vi "Main.vi"(11 "Module Admin":refnum<class "Delacor_lib_QMH_Cloneable Module Admin.lvclass">) -> ()   [LabVIEW 2020, in "Arduino-Adafruit stepper.lvlib"]
doc: "This template is based off of the Queued Message Handler design pattern and the Queued Message Handler project template that ships with LabVIEW.\n\nThe main difference is that the queue is private to this module and communication between modules is performed via Broadcast and Request events.\n\nRequest events are wrapped in public API methods and are handled in the Event Handling Loop (EHL) of this VI. Any module can register for Broadcast events sent by this module. The EHL generates messages based on user interface actions.\n\nThe Message Handling Loop (MHL) processes messages generated by the EHL, or by other messages. The messages are string values, so new messages can be added easily to the Message Cases case structure in the MHL. Each message cluster can also provide an optional value for Message Data, which is a variant that can be converted to whatever message-specific data is required.\n_____\nBased on DQMH Project Template 7.0.1.1316."
uses:
  Arduino-Adafruit stepper.lvlib
  <vilib>/Delacor/Delacor QMH/Libraries/Cloneable Module Admin_class/Delacor_lib_QMH_Cloneable Module Admin.lvclass
  C:/Program Files (x86)/National Instruments/LabVIEW 2020/vi.lib/Delacor/Delacor QMH/Libraries/Module Admin_class/Delacor_lib_QMH_Module Admin.lvclass
  Module Data--cluster.ctl
  <vilib>/Delacor/Delacor QMH/Libraries/Cloneable Module Admin_class/Delacor_lib_QMH_Cloneable Module Admin.lvclass/Delacor_lib_QMH_Cloneable Module Admin.ctl
  Stop Argument--cluster.ctl
  <vilib>/Delacor/Delacor QMH/Libraries/Message Queue_class/Delacor_lib_QMH_Message Queue.lvclass/Delacor_lib_QMH_Message Queue.ctl
  <vilib>/Delacor/Delacor QMH/Libraries/Module Admin_class/Delacor_lib_QMH_Module Admin.lvclass/Delacor_lib_QMH_Module Admin.ctl
  Connect Argument--cluster.ctl
  Arduino stepper library/Public/Controls/Com Port Options.ctl
  Disconnect Argument--cluster.ctl
  Init motors Argument--cluster.ctl
  Arduino stepper library/Public/Controls/Motor initialization parameters--cluster.ctl
  Home motors Argument--cluster.ctl
  Arduino stepper library/Public/Controls/Motor direction.ctl
  <vilib>/Utility/miscctls.llb/LVPointTypeDef.ctl
  <vilib>/Instr/_visa.llb/VISA Flush IO Buffer Mask.ctl
  <vilib>/Instr/_visa.llb/VISA Set IO Buffer Mask.ctl
  <vilib>/Delacor/Delacor QMH/Libraries/Cloneable Module Admin_class/Delacor_lib_QMH_Get Module ID.vi
  <vilib>/Delacor/Delacor QMH/Libraries/Message Queue_class/Delacor_lib_QMH_Enqueue Message (Single).vi
  <vilib>/Delacor/Delacor QMH/Libraries/Module Admin_class/Delacor_lib_QMH_Get External Launch.vi
  <vilib>/Instr/_visa.llb/VISA Configure Serial Port (Instr).vi
  <vilib>/Delacor/Delacor QMH/Libraries/Message Queue_class/Delacor_lib_QMH_Message Queue.lvclass
  Arduino stepper library/Control de MaP.lvlib
panel:
  out "error out":errorcluster
  out "Status":string
  # "Other processes communicate with this Module via its Public API (wrappers for its Request Events).\n\nThis Module communicates with other processes via its Broadcast Events.\nAny process that wants to receive these messages can register for this module's Broadcast events."
  # "This template is for the DQMH framework. See the block diagram for more information on how to use this template."
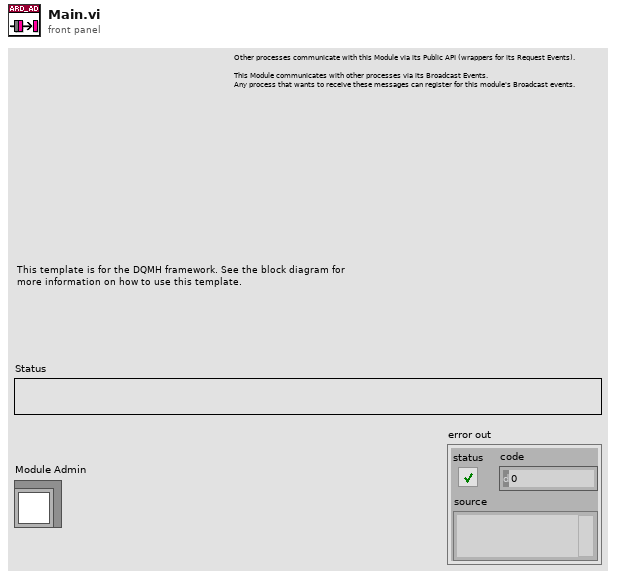
[diagram p1: front panel]
types:
  T1 = typedef "Arduino-Adafruit stepper.lvlib/Request Events--cluster.ctl" = cluster{"Stop Module":refnum<user-event>, "Show Panel":refnum<user-event>, "Hide Panel":refnum<user-event>, "Show Diagram":refnum<user-event>, "Get Module Execution Status":refnum<user-event>, "Initialize Arduino":refnum<user-event>, "Connect":refnum<user-event>, "Disconnect":refnum<user-event>, "Init motors":refnum<user-event>, "Home motors":refnum<user-event>}
  T2 = typedef "Arduino-Adafruit stepper.lvlib/Module Data--cluster.ctl" = cluster{"Status":string, "VISA resource":refnum<visa-resource-name>, "Connected?":bool}
  T3 = enum32{"invalid lock state", "Not Locked", "Locked (No Password)", "Password-protected"}
  T4 = typedef "Arduino-Adafruit stepper.lvlib/Stop Argument--cluster.ctl" = cluster{"Module ID":i32, "Origin":string, "Exit via Stop Module Req?":bool, "Wait for Module to stop?":bool}
  T5 = typedef "Arduino-Adafruit stepper.lvlib/Connect Argument--cluster.ctl" = cluster{"Module ID":i32, "VISA resource":refnum<visa-resource-name>, "COM options":T6}
  T6 = typedef "Control de MaP.lvlib/Com Port Options.ctl" = cluster{"baud rate":u32, "data bits":u16, "parity":enum16{"None", "Odd", "Even", "Mark", "Space"}}
  T7 = typedef "Arduino-Adafruit stepper.lvlib/Disconnect Argument--cluster.ctl" = cluster{"Module ID":i32, "Boolean":bool}
  T8 = typedef "Arduino-Adafruit stepper.lvlib/Init motors Argument--cluster.ctl" = cluster{"Module ID":i32, "Comando":T9}
  T9 = typedef "Control de MaP.lvlib/Motor initialization parameters--cluster.ctl" = cluster{"Action":u8, "Steps per rev motor 1":u8, "Steps per rev motor 2":u8, "RPM motor 1":u16, "RPM motor 2":u16}
  T10 = typedef "Arduino-Adafruit stepper.lvlib/Home motors Argument--cluster.ctl" = cluster{"Module ID":i32, "Home direction (M1)":T11, "Home direction (M2)":T11}
  T11 = typedef "Control de MaP.lvlib/Motor direction.ctl" = u8
  T12 = typedef "LVPointTypeDef.ctl" = cluster{"Horizontal":i16, "Vertical":i16}
  T13 = enum32{"Invalid", "Standard", "Closed", "Hidden", "Minimized", "Maximized"}
  T14 = typedef "VISA Set IO Buffer Mask.ctl" = u16
  T15 = typedef "VISA Flush IO Buffer Mask.ctl" = u16
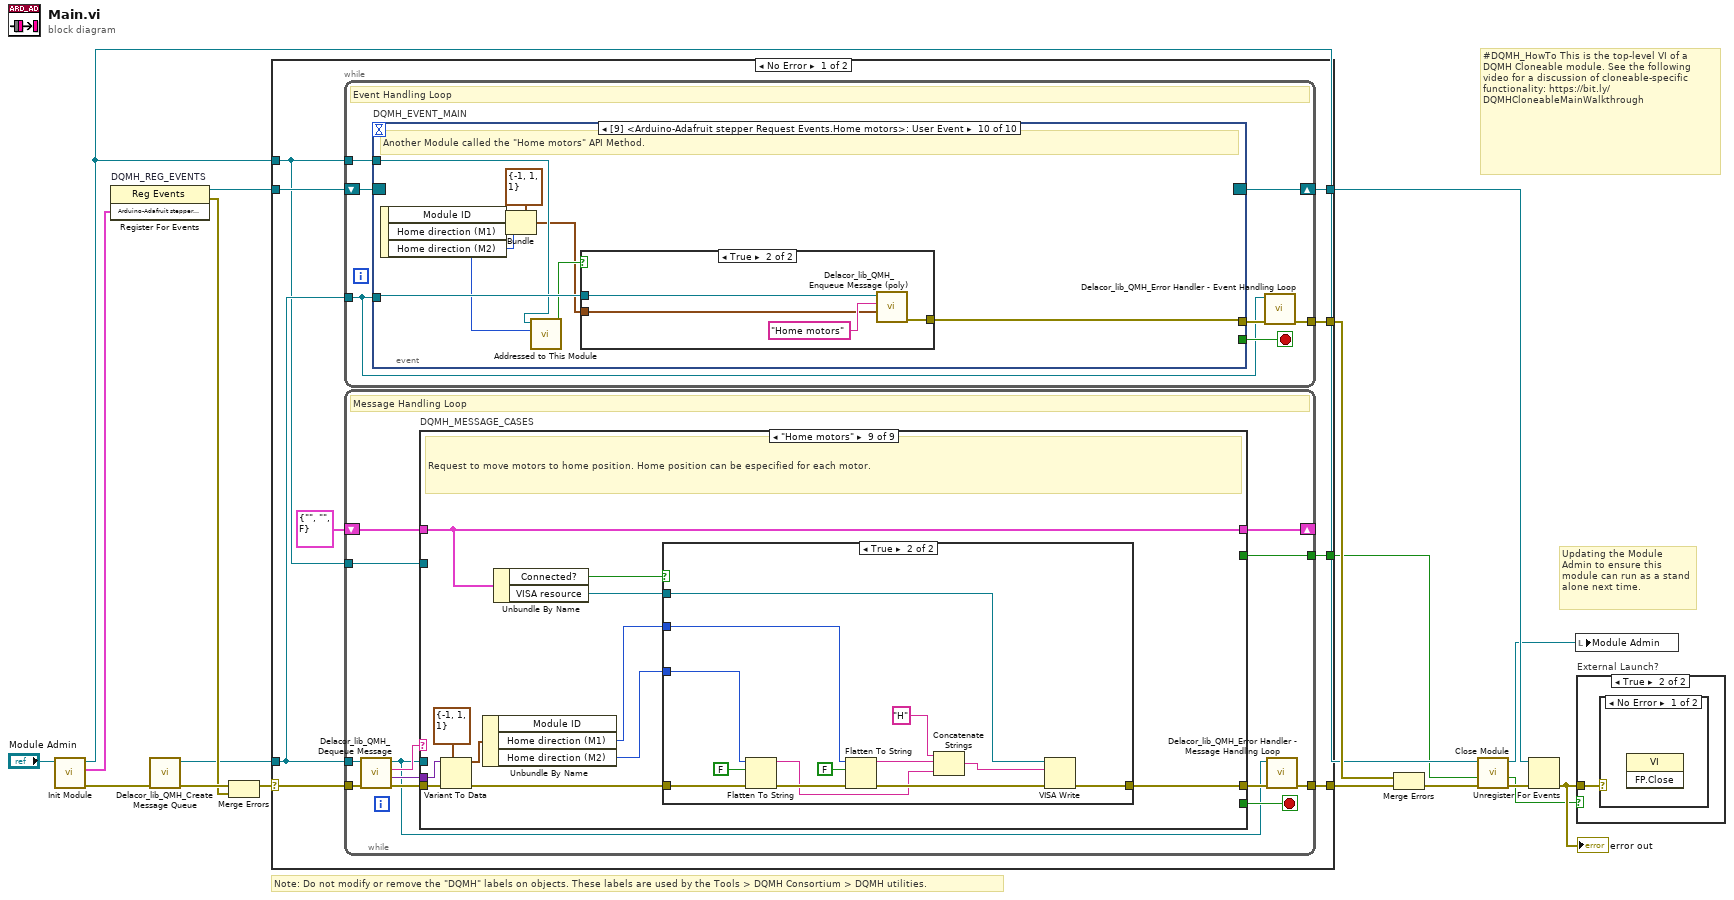
[diagram p0: block diagram]
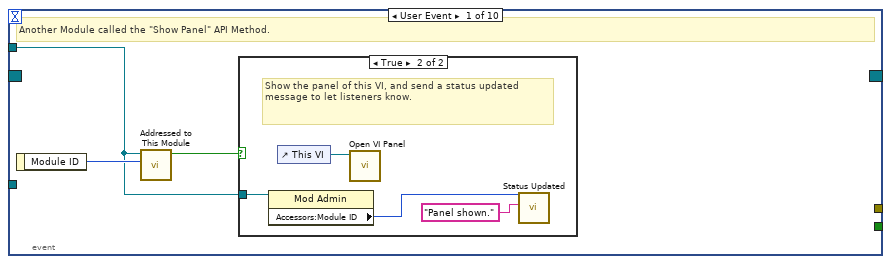
[diagram p2: hidden frame]
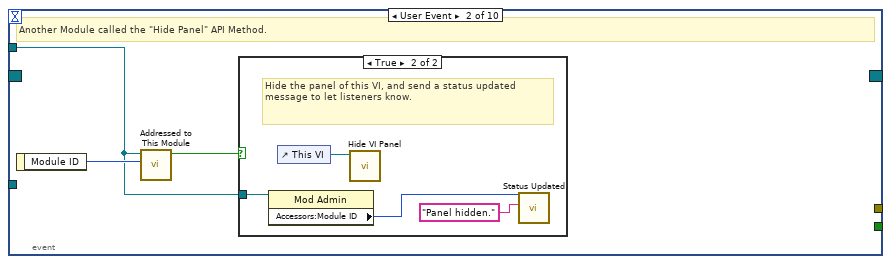
[diagram p4: hidden frame]
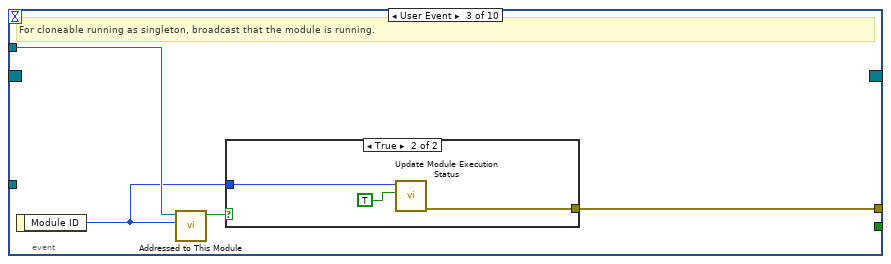
[diagram p6: hidden frame]
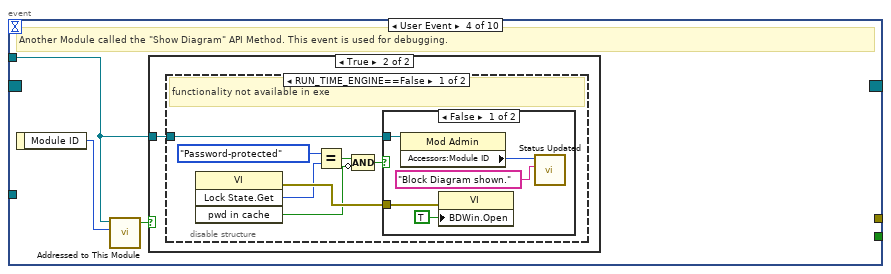
[diagram p8: hidden frame]
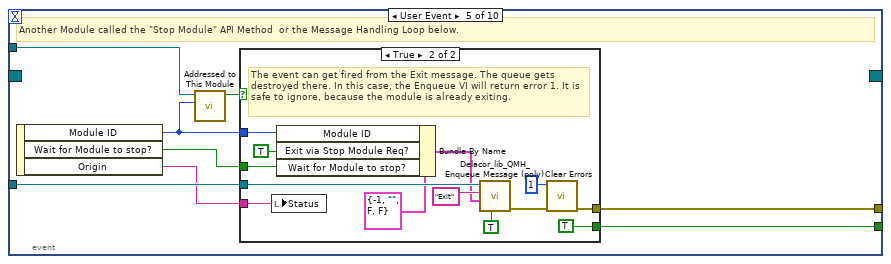
[diagram p12: hidden frame]
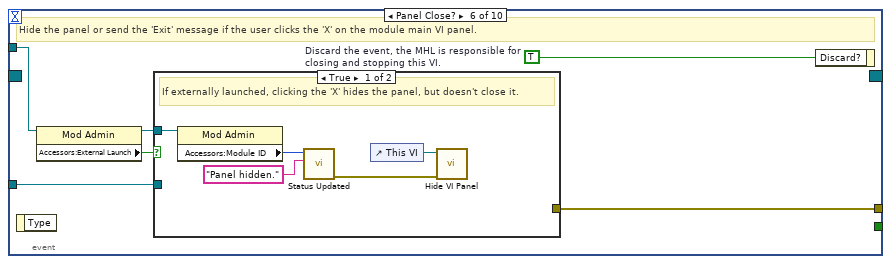
[diagram p14: hidden frame]
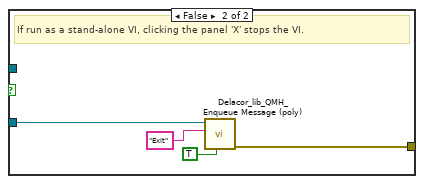
[diagram p15: hidden frame]
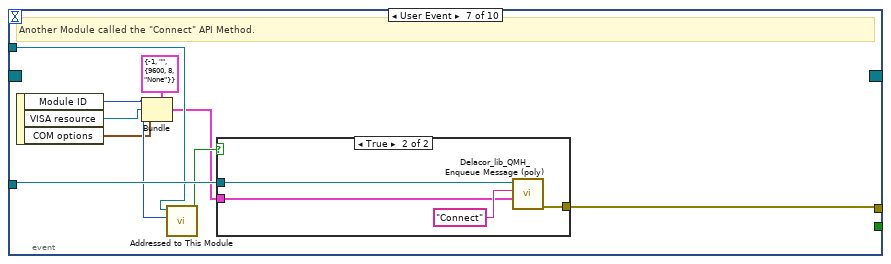
[diagram p16: hidden frame]
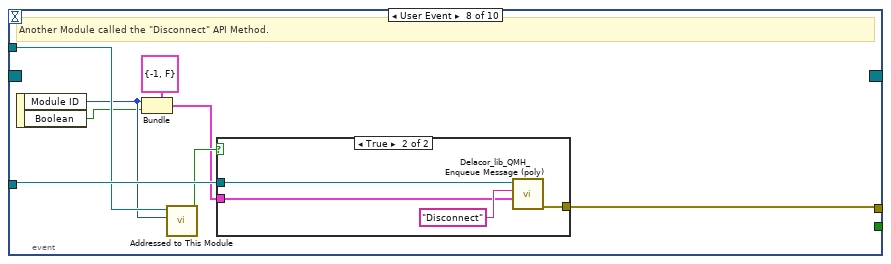
[diagram p18: hidden frame]
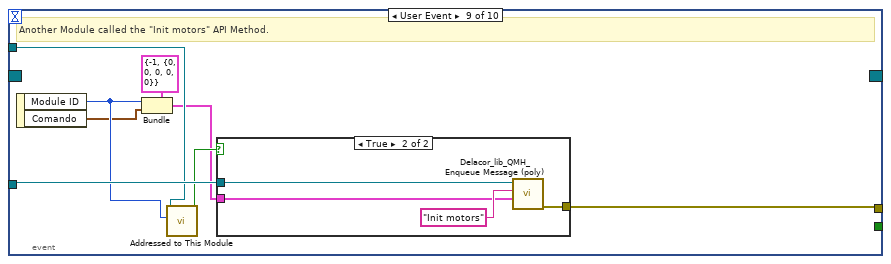
[diagram p20: hidden frame]
diagram:
  # "#DQMH_HowTo This is the top-level VI of a DQMH Cloneable module. See the following video for a discussion of cloneable-specific functionality: https://bit.ly/DQMHCloneableMainWalkthrough"
  # "Note: Do not modify or remove the \"DQMH\" labels on objects. These labels are used by the Tools > DQMH Consortium > DQMH utilities."
  # "Updating the Module Admin to ensure this module can run as a stand alone next time."
  n1 = call "Init Module.vi"("Cloneable Module Admin in"="Module Admin") -> ("error out"=w15:errorcluster, "Arduino-Adafruit stepper Request Events"=w7:T1, "Cloneable Module Admin out"=w4:refnum<class "Delacor_lib_QMH_Cloneable Module Admin.lvclass">)  [unwired: 8 in]
  n2 = register-events "DQMH_REG_EVENTS"(w7) -> (reference out=w8:refnum<event-registration>, error out=w10:errorcluster)  [unwired: 2 in]
  n3 = call <vilib>:"Delacor_lib_QMH_Create Message Queue.vi"("error in"=w15) -> ("error out"=w12:errorcluster, "Message Queue"=w6:refnum<class "Delacor_lib_QMH_Message Queue.lvclass">)  [unwired: 9 in]
  n4 = Merge Errors(w12, w10) -> (w11:errorcluster)
  n5 = case shown="No Error" w11 {
    selector: w11 -> [w25 w401]
    tunnel: [w27 w400] -> w16
    tunnel: [w24 w399] -> w9
    tunnel: w8 -> [w22 w399]
    tunnel: w6 -> [w21 w392]
    tunnel: [w26 _] -> w17
    tunnel: w4 -> [w20 w395]
    tunnel: [w19 _] -> w2
    frame No Error {
      n6 = while {
        tunnel: w21 -> [w28]
        shift-right: [w31] -> w24
        shift-left: w22 -> [w32]
        tunnel: [w33] -> w26
        tunnel: w20 -> [w29]
        stop <- w30 stop-if-true
        # "Event Handling Loop"
        n7 = event "DQMH_EVENT_MAIN" shown="[9] <Arduino-Adafruit stepper Request Events.Home motors>: User Event" {
          selector: w32 -> [_ _ _ _ _ _ _ _ _ _]
          dyn-events: [_ _ _ _ _ _ _ _ _ _] -> w31
          timeout: _ -> [_ _ _ _ _ _ _ _ _ _]
          tunnel: [_ _ _ _ w75 _ _ _ _ _] -> w30
          tunnel: w28 -> [_ _ _ _ w78 w95 w116 w128 w140 w153]
          tunnel: [_ _ w52 _ w79 w98 w108 w121 w134 w145] -> w34
          tunnel: w29 -> [w35 w42 w50 w56 w77 w96 w114 w126 w138 w151]
          event User Event {
            # "Another Module called the \"Show Panel\" API Method."
            n8 = event-data() -> ("Module ID"=w36:i32)  [unwired: 1 in]
            n9 = call "Addressed to This Module.vi"("Module ID from Argument"=w36, "Module Admin"=w35) -> ("Addressed to this instance?"=w37:bool)  [unwired: 8 in, 1 out]
            n10 = case shown="True" w37 {
              tunnel: w35 -> [_ w39]
              frame False {
              }
              frame True {
                # "Show the panel of this VI, and send a status updated message to let listeners know."
                n11 = property on="Property Node" class="Mod Admin"(reference=w39) -> ("Accessors:Module ID"=w38:i32)  [unwired: 1 in, 2 out]
                n12 = control-ref of="This VI"() -> (w41:refnum<vi>)
                n13 = call "Open VI Panel.vi"("VI"=w41) -> ()  [unwired: 10 in, 1 out]
                n14 = call "Status Updated.vi"("Status"="Panel shown." ("format string"), "Module ID"=w38) -> ()  [unwired: 9 in, 1 out]
              }
            }
          }
          event User Event {
            # "Another Module called the \"Hide Panel\" API Method."
            n15 = event-data() -> ("Module ID"=w43:i32)  [unwired: 1 in]
            n16 = call "Addressed to This Module.vi"("Module ID from Argument"=w43, "Module Admin"=w42) -> ("Addressed to this instance?"=w44:bool)  [unwired: 8 in, 1 out]
            n17 = case shown="True" w44 {
              tunnel: w42 -> [_ w46]
              frame False {
              }
              frame True {
                # "Hide the panel of this VI, and send a status updated message to let listeners know."
                n18 = property on="Property Node" class="Mod Admin"(reference=w46) -> ("Accessors:Module ID"=w45:i32)  [unwired: 1 in, 2 out]
                n19 = control-ref of="This VI"() -> (w48:refnum<vi>)
                n20 = call "Hide VI Panel.vi"("VI"=w48) -> ()  [unwired: 10 in, 1 out]
                n21 = call "Status Updated.vi"("Status"="Panel hidden." ("format string"), "Module ID"=w45) -> ()  [unwired: 9 in, 1 out]
              }
            }
          }
          event User Event {
            # "For cloneable running as singleton, broadcast that the module is running."
            n22 = event-data() -> ("Module ID"=w49:i32)  [unwired: 1 in]
            n23 = call "Addressed to This Module.vi"("Module ID from Argument"=w49, "Module Admin"=w50) -> ("Addressed to this instance?"=w51:bool)  [unwired: 8 in, 1 out]
            n24 = case shown="True" w51 {
              tunnel: [_ w55] -> w52
              tunnel: w49 -> [_ w54]
              frame False {
              }
              frame True {
                n25 = call "Update Module Execution Status.vi"("Running?"=TRUE, "Module ID"=w54) -> ("error out"=w55:errorcluster)  [unwired: 9 in]
              }
            }
          }
          event User Event {
            # "Another Module called the \"Show Diagram\" API Method. This event is used for debugging."
            n26 = event-data() -> ("Module ID"=w57:i32)  [unwired: 1 in]
            n27 = call "Addressed to This Module.vi"("Module ID from Argument"=w57, "Module Admin"=w56) -> ("Addressed to this instance?"=w58:bool)  [unwired: 8 in, 1 out]
            n28 = case shown="True" w58 {
              tunnel: w56 -> [_ w59]
              frame False {
              }
              frame True {
                n29 = disable-structure shown="RUN_TIME_ENGINE==False" {
                  disable-tunnel: w59 -> [w60 _]
                  frame condition #0 (active) {
                    # "functionality not available in exe"
                    n30 = invoke on="Invoke Node" class="VI" method="Lock State.Get"() -> (error out=w66:errorcluster, "Get Lock State"=w65:T3, "pwd in cache"=w62:bool)  [unwired: 4 in, 1 out]
                    n31 = Equal?(x=T3."Password-protected", y=w65) -> (x = y?=w63:bool)
                    n32 = Compound Arithmetic op=AND(w63, invert w62) -> (w61:bool)
                    n33 = case shown="False" w61 {
                      tunnel: w66 -> [w71 _]
                      tunnel: w60 -> [w68 _]
                      frame False {
                        n34 = property on="Property Node" class="Mod Admin"(reference=w68) -> ("Accessors:Module ID"=w67:i32)  [unwired: 1 in, 2 out]
                        n35 = property on="Property Node" class="VI"(error in=w71, "BDWin.Open"=TRUE ("Block Diagram Window:Open")) -> ()  [unwired: 1 in, 2 out]
                        n36 = call "Status Updated.vi"("Status"="Block Diagram shown." ("format string"), "Module ID"=w67) -> ()  [unwired: 9 in, 1 out]
                      }
                      frame True {
                        # "Password-protected VI, and the password is not in the cache. Do not show the diagram."
                      }
                    }
                  }
                  frame condition #1 {
                  }
                }
              }
            }
          }
          event User Event {
            # "Another Module called the \"Stop Module\" API Method  or the Message Handling Loop below."
            n37 = event-data() -> ("Module ID"=w73:i32, "Wait for Module to stop?"=w74:bool, "Origin"=w72:string)  [unwired: 1 in]
            n38 = call "Addressed to This Module.vi"("Module ID from Argument"=w73, "Module Admin"=w77) -> ("Addressed to this instance?"=w76:bool)  [unwired: 8 in, 1 out]
            n39 = case shown="True" w76 {
              tunnel: [_ w91] -> w79
              tunnel: w78 -> [_ w87]
              tunnel: [_ TRUE] -> w75
              tunnel: w74 -> [_ w82]
              tunnel: w73 -> [_ w84]
              tunnel: w72 -> [_ w80]
              frame False {
              }
              frame True {
                # "The event can get fired from the Exit message. The queue gets destroyed there. In this case, the Enqueue VI will return error 1. It is safe to ignore, because the module is already exiting."
                n40 = local write "Status"(w80) -> ()
                n41 = Bundle By Name(cluster=T4 {"Module ID"=-1, "Origin"="", "Exit via Stop Module Req?"=FALSE, "Wait for Module to stop?"=FALSE} ("Stop Argument"), "Module ID"=w84, "Exit via Stop Module Req?"=TRUE, "Wait for Module to stop?"=w82) -> (w81:T4)
                n42 = call-poly <vilib>:"Delacor_lib_QMH_Enqueue Message (poly).vi"("Priority Message? (F)"=TRUE, "Message Data"=w81, "Message"="Exit", "Message Queue in"=w87) -> ("error out"=w92:errorcluster)  [unwired: 6 in, 1 out]
                n43 = call <vilib>:"Clear Errors.vi"("error in (no error)"=w92, "specific error code to clear (0: all)"=1) -> ("error out"=w91:errorcluster)  [unwired: 4 in, 1 out]
              }
            }
          }
          event Panel Close? {
            w97 = TRUE  # Discard the event, the MHL is responsible for closing and stopping this VI.
            # "Hide the panel or send the 'Exit' message if the user clicks the 'X' on the module main VI panel."
            n44 = event-data() -> ()  [unwired: 1 in, 1 out]
            n45 = property on="Property Node" class="Mod Admin"(reference=w96) -> (reference out=w93:refnum<class "Delacor_lib_QMH_Cloneable Module Admin.lvclass">, "Accessors:External Launch"=w94:bool)  [unwired: 1 in, 1 out]
            n46 = case shown="True" w94 {
              tunnel: w95 -> [_ w106]
              tunnel: [_ w107] -> w98
              tunnel: w93 -> [w101 _]
              frame True {
                # "If externally launched, clicking the 'X' hides the panel, but doesn't close it."
                n47 = property on="Property Node" class="Mod Admin"(reference=w101) -> ("Accessors:Module ID"=w100:i32)  [unwired: 1 in, 2 out]
                n48 = call "Status Updated.vi"("Status"="Panel hidden." ("format string"), "Module ID"=w100) -> ("error out"=w99:errorcluster)  [unwired: 9 in]
                n49 = control-ref of="This VI"() -> (w103:refnum<vi>)
                n50 = call "Hide VI Panel.vi"("error in"=w99, "VI"=w103) -> ()  [unwired: 9 in, 1 out]
              }
              frame False {
                # "If run as a stand-alone VI, clicking the panel 'X' stops the VI."
                n51 = call-poly <vilib>:"Delacor_lib_QMH_Enqueue Message (poly).vi"("Priority Message? (F)"=TRUE, "Message"="Exit", "Message Queue in"=w106) -> ("error out"=w107:errorcluster)  [unwired: 7 in, 1 out]
              }
            }
            n52 = event-data ("Event Filter Node")("Discard?"=w97) -> ()  [unwired: 1 in, 1 out]
          }
          event User Event {
            # "Another Module called the \"Connect\" API Method."
            n53 = event-data() -> ("Module ID"=w111:i32, "VISA resource"=w110:refnum<visa-resource-name>, "COM options"=w109:T6)  [unwired: 1 in]
            n54 = Bundle(cluster=T5 {"Module ID"=-1, "VISA resource"="", "COM options"={"baud rate"=9600, "data bits"=8, "parity"=enum."None"}} ("Connect Argument"), "Module ID"=w111, "VISA resource"=w110, "COM options"=w109) -> (w112:T5)
            n55 = call "Addressed to This Module.vi"("Module ID from Argument"=w111, "Module Admin"=w114) -> ("Addressed to this instance?"=w115:bool)  [unwired: 8 in, 1 out]
            n56 = case shown="True" w115 {
              tunnel: w116 -> [_ w120]
              tunnel: w112 -> [_ w118]
              tunnel: [_ w117] -> w108
              frame False {
              }
              frame True {
                n57 = call-poly <vilib>:"Delacor_lib_QMH_Enqueue Message (poly).vi"("Message Data"=w118, "Message"="Connect", "Message Queue in"=w120) -> ("error out"=w117:errorcluster)  [unwired: 7 in, 1 out]
              }
            }
          }
          event User Event {
            # "Another Module called the \"Disconnect\" API Method."
            n58 = event-data() -> ("Module ID"=w123:i32, "Boolean"=w122:bool)  [unwired: 1 in]
            n59 = Bundle(cluster=T7 {"Module ID"=-1, "Boolean"=FALSE} ("Disconnect Argument"), "Module ID"=w123, "Boolean"=w122) -> (w124:T7)
            n60 = call "Addressed to This Module.vi"("Module ID from Argument"=w123, "Module Admin"=w126) -> ("Addressed to this instance?"=w127:bool)  [unwired: 8 in, 1 out]
            n61 = case shown="True" w127 {
              tunnel: w128 -> [_ w132]
              tunnel: w124 -> [_ w130]
              tunnel: [_ w129] -> w121
              frame False {
              }
              frame True {
                n62 = call-poly <vilib>:"Delacor_lib_QMH_Enqueue Message (poly).vi"("Message Data"=w130, "Message"="Disconnect", "Message Queue in"=w132) -> ("error out"=w129:errorcluster)  [unwired: 7 in, 1 out]
              }
            }
          }
          event User Event {
            # "Another Module called the \"Init motors\" API Method."
            n63 = event-data() -> ("Module ID"=w135:i32, "Comando"=w133:T9)  [unwired: 1 in]
            n64 = Bundle(cluster=T8 {"Module ID"=-1, "Comando"={"Action"=0, "Steps per rev motor 1"=0, "Steps per rev motor 2"=0, "RPM motor 1"=0, "RPM motor 2"=0}} ("Init motors Argument"), "Module ID"=w135, "Comando"=w133) -> (w136:T8)
            n65 = call "Addressed to This Module.vi"("Module ID from Argument"=w135, "Module Admin"=w138) -> ("Addressed to this instance?"=w139:bool)  [unwired: 8 in, 1 out]
            n66 = case shown="True" w139 {
              tunnel: w140 -> [_ w144]
              tunnel: w136 -> [_ w142]
              tunnel: [_ w141] -> w134
              frame False {
              }
              frame True {
                n67 = call-poly <vilib>:"Delacor_lib_QMH_Enqueue Message (poly).vi"("Message Data"=w142, "Message"="Init motors", "Message Queue in"=w144) -> ("error out"=w141:errorcluster)  [unwired: 7 in, 1 out]
              }
            }
          }
          event User Event {
            # "Another Module called the \"Home motors\" API Method."
            n68 = event-data() -> ("Module ID"=w148:i32, "Home direction (M1)"=w147:T11, "Home direction (M2)"=w146:T11)  [unwired: 1 in]
            n69 = Bundle(cluster=T10 {"Module ID"=-1, "Home direction (M1)"=1, "Home direction (M2)"=1} ("Home motors Argument"), "Module ID"=w148, "Home direction (M1)"=w147, "Home direction (M2)"=w146) -> (w149:T10)
            n70 = call "Addressed to This Module.vi"("Module ID from Argument"=w148, "Module Admin"=w151) -> ("Addressed to this instance?"=w152:bool)  [unwired: 8 in, 1 out]
            n71 = case shown="True" w152 {
              tunnel: w153 -> [_ w157]
              tunnel: w149 -> [_ w155]
              tunnel: [_ w154] -> w145
              frame False {
              }
              frame True {
                n72 = call-poly <vilib>:"Delacor_lib_QMH_Enqueue Message (poly).vi"("Message Data"=w155, "Message"="Home motors", "Message Queue in"=w157) -> ("error out"=w154:errorcluster)  [unwired: 7 in, 1 out]
              }
            }
          }
        }
        n73 = call-dynamic "Delacor_lib_QMH_Error Handler - Event Handling Loop.vi"("error in"=w34, "Message Queue in"=w28) -> ("dup error in"=w33:errorcluster)  [unwired: 8 in, 1 out]
      }
      n74 = while {
        tunnel: w21 -> [w158]
        shift-right: [w165] -> _
        shift-left: T2 {"Status"="", "VISA resource"="", "Connected?"=FALSE} ("Data Cluster") -> [w166]
        tunnel: w25 -> [w169]
        tunnel: [w167] -> w27
        tunnel: w20 -> [w160]
        tunnel: [w159] -> w19
        stop <- w164 stop-if-true
        # "Message Handling Loop"
        n75 = call-dynamic "Delacor_lib_QMH_Dequeue Message.vi"("error in"=w169, "Message Queue in"=w158) -> ("error out"=w168:errorcluster, "Message Data"=w162:variant, "Message"=w163:string, "Message Queue out"=w161:refnum<class "Delacor_lib_QMH_Message Queue.lvclass">)  [unwired: 6 in]
        n76 = case "DQMH_MESSAGE_CASES" shown="\"Home motors\"" w163 {
          selector: w163 -> [_ _ _ _ _ w290 _ _ _]
          tunnel: w161 -> [_ _ _ w250 w283 _ _ _ _]
          tunnel: w168 -> [w189 w207 w247 w259 w288 w299 w310 w336 w377]
          tunnel: [w187 w192 w247 w255 w284 w300 w302 w326 w367] -> w170
          tunnel: w166 -> [w180 w198 w246 w254 w271 w297 w306 w332 w373]
          tunnel: [w179 w197 w246 w254 w271 w297 w306 w332 w373] -> w165
          tunnel: [_ _ _ _ w282 _ _ _ _] -> w164
          tunnel: w162 -> [_ w206 _ w253 w280 _ w309 w335 w376]
          tunnel: w160 -> [w174 _ _ w252 w275 w296 _ _ _]
          tunnel: [_ _ _ _ w278 _ _ _ _] -> w159
          frame "Initialize" {
            w171 = "Initial Message" ("Initial Message")
            # "#CodeNeeded - Initialize the appearance of the front panel."
            # "#CodeNeeded - Initialize your state data here."
            # "Initialize - Any operation that needs to be done before the module can receive messages. Synchronize Caller Events.vi will inform Start Module.vi that the module has launched and is ready to receive messages. Module Did Init.vi will broadcast that the module initialized."
            n77 = call "Synchronize Caller Events.vi"("error in"=w189, "Module Admin"=w174) -> ("error out"=w188:errorcluster, "Module Admin out"=w173:refnum<class "Delacor_lib_QMH_Cloneable Module Admin.lvclass">)  [unwired: 8 in]
            n78 = property on="Property Node" class="Mod Admin"(reference=w173) -> ("Accessors:Module ID"=w176:i32, "Accessors:External Launch"=w175:bool)  [unwired: 1 in, 2 out]
            n79 = call "Module Name--constant.vi"("Module ID"=w176) -> ("Module Name"=w184:string)  [unwired: 10 in]
            n80 = property on="Property Node" class="VI"("Front Panel.Title"=w184) -> (reference out=w186:refnum<vi>, error out=w191:errorcluster)  [unwired: 2 in]
            n81 = Select(t=T13."Hidden" ("State"), s=w175, f=T13."Standard" ("State")) -> (s? t:f=w181:T13)
            n82 = invoke on="Invoke Node" class="VI" method="FP.Open"(reference=w186, error in=w191, "State"=w181) -> (reference out=w185:refnum<vi>, error out=w190:errorcluster)  [unwired: 2 in, 3 out]
            n83 = call "Module Name--constant.vi"("Module ID"=w176) -> ("Module Name"=w177:string)  [unwired: 10 in]
            n84 = Bundle By Name(cluster=w180, "Status"=w171) -> (w179:T2)
            n85 = invoke on="Invoke Node" class="VI" method="FP.Center"(reference=w185, error in=w190) -> ()  [unwired: 1 in, 3 out]
            n86 = property on="Pane" class="Pane"("Origin"=T12 {"Horizontal"=0, "Vertical"=0}) -> ()  [unwired: 2 in, 2 out]
            n87 = call "Module Did Init.vi"("error in"=w188, "Initialized?"=TRUE, "Origin"=w177, "Module ID"=w176) -> ("error out"=w187:errorcluster)  [unwired: 7 in]
            "Status" <- w171
          }
          frame "Connect" {
            # "Request to connect to Arduino. After connection tries, broadcasts either a successful or failed connection status."
            n88 = Variant To Data(error in=w207, type=T5 {"Module ID"=-1, "VISA resource"="", "COM options"={"baud rate"=9600, "data bits"=8, "parity"=enum."None"}} ("Connect Argument"), Variant=w206) -> (data=w204:T5, error out=w199:errorcluster)
            n89 = Unbundle By Name(w204) -> ("Module ID"=w193:i32, "VISA resource"=w202:refnum<visa-resource-name>, "COM options"=w203:T6)
            n90 = VISA Open(error in (no error)=w199, VISA resource name=w202) -> (VISA resource name=w201:refnum<visa-resource-name>, error out=w200:errorcluster)  [unwired: 3 in]
            n91 = case shown="No Error" w200 {
              selector: w200 -> [_ w238 w243]
              tunnel: [w217 w240 w245] -> w196
              tunnel: [w219 w239 w241] -> w195
              tunnel: w203 -> [w234 _ _]
              tunnel: w201 -> [w221 w240 w245]
              tunnel: [w216 _ _] -> w194
              frame No Error {
                w222 = u32 1024  # Buffer size
                w223 = T14 32 items=["I/O Receive Buffer"=16, "I/O Transmit Buffer"=32, "I/O Receive and Transmit Buffer"=48] ("Mask")
                w224 = T15 16 items=["Flush Receive Buffer"=16, "Write Transmit Buffer to Device"=32, "Flush Receive Buffer (No I/O)"=64, "Flush Transmit Buffer"=128] ("Mask")
                w226 = T15 128 items=["Flush Receive Buffer"=16, "Write Transmit Buffer to Device"=32, "Flush Receive Buffer (No I/O)"=64, "Flush Transmit Buffer"=128] ("Mask")
                n92 = Unbundle By Name(w234) -> ("baud rate"=w233:u32, "data bits"=w232:u16, "parity"=w231:enum16{"None", "Odd", "Even", "Mark", "Space"})
                n93 = call-poly "VISA Configure Serial Port"("VISA resource name"=w221, "baud rate (9600)"=w233, "data bits (8)"=w232, "parity (0:none)"=w231) -> ("VISA resource name out"=w230:refnum<visa-resource-name>, "error out"=w228:errorcluster)  [unwired: 10 in]
                n94 = VISA Set I/O Buffer Size(VISA resource name=w230, mask (16)=w223, size (4096)=w222, error in (no error)=w228) -> (VISA resource name out=w229:refnum<visa-resource-name>, error out=w227:errorcluster)
                n95 = Or(x=w226, y=w224) -> (x .or. y?=w225:T15)
                n96 = VISA Flush I/O Buffer(VISA resource name=w229, mask (16)=w225, error in (no error)=w227) -> (VISA resource name out=w218:refnum<visa-resource-name>, error out=w220:errorcluster)
                n97 = call "Validate connection.vi"("error in (no error)"=w220, "VISA Refnum in"=w218) -> ("error out"=w219:errorcluster, "Connection valid?"=w216:bool, "VISA Refnum out"=w217:refnum<visa-resource-name>)  [unwired: 7 in]
              }
              frame Default {
                n98 = Unbundle By Name(w238) -> ("code"=w236:i32)
                n99 = Format Into String(initial string="Error no manejado. Código de error: %d.", w236) -> (resulting string=w235:string)  [unwired: 2 in, 1 out]
                n100 = call <vilib>:"Clear Errors.vi"("error in (no error)"=w238) -> ("error out"=w239:errorcluster)  [unwired: 5 in, 1 out]
                n101 = One Button Dialog(message=w235) -> ()  [unwired: 1 in, 1 out]
              }
              frame Error {
                n102 = call <vilib>:"Clear Errors.vi"("error in (no error)"=w243, "specific error code to clear (0: all)"=-1073807343) -> ("error out"=w241:errorcluster)  [unwired: 4 in, 1 out]
                n103 = One Button Dialog(message="No se ha encontrado el Arduino. Por favor, verifique la  conexión y vuelva a intentarlo.") -> ()  [unwired: 1 in, 1 out]
              }
            }
            n104 = case shown="True" w194 {
              tunnel: w195 -> [w211 w215]
              tunnel: w193 -> [w209 w214]
              tunnel: [w210 w213] -> w192
              frame False {
                n105 = call "Connection failed.vi"("error in"=w211, "Connected?"=FALSE, "Module ID"=w209) -> ("error out"=w210:errorcluster)  [unwired: 8 in]
              }
              frame True {
                n106 = call "Connection successful.vi"("error in"=w215, "Connected?"=TRUE, "Module ID"=w214) -> ("error out"=w213:errorcluster)  [unwired: 8 in]
              }
            }
            n107 = Bundle By Name(cluster=w198, "Connected?"=w194, "VISA resource"=w196) -> (w197:T2)
          }
          frame "---Exit and Error Handling---" {
            # "Separator - the following cases handle errors and exit messages."
          }
          frame "Error" {
            # "#CodeRecommended - If the module is running in standalone mode (External Launch = FALSE), this code will pop up an error dialog and call the 'Exit' message if an error occurs. Add more fine-grained error management here."
            # "Error - Check the error message data and respond accordingly. This message is sent by the \"Error Handler\" VIs at the end of each loop in this application."
            n108 = property on="Property Node" class="Mod Admin"(reference=w252) -> ("Accessors:External Launch"=w251:bool, "Accessors:Module ID"=w249:i32)  [unwired: 1 in, 2 out]
            n109 = Variant To Data(error in=w259, type=errorcluster {"status"=FALSE, "code"=0, "source"=""} ("error constant"), Variant=w253) -> (data=w248:errorcluster, error out=w257:errorcluster)
            n110 = local write "error out"(w248) -> ()
            n111 = call "Error Reported.vi"("Error"=w248, "Module ID"=w249) -> ()  [unwired: 9 in, 1 out]
            n112 = case shown="False" w251 {
              tunnel: [w264 _] -> w256
              tunnel: w250 -> [w262 _]
              tunnel: w248 -> [w263 _]
              frame False {
                n113 = disable-structure shown="Default" {
                  disable-tunnel: w263 -> [w265 _]
                  frame condition #0 (active) {
                    # "If the module is running standalone, then pop up an error dialog and call the \"Exit\" message."
                    n114 = call <vilib>:"Simple Error Handler.vi"("error in (no error)"=w265) -> ()  [unwired: 4 in, 5 out]
                  }
                  frame condition #1 {
                    # "To prevent the Simple Error Handler VI from being loaded (e.g. when deploying to a Real-Time target), add the Conditional Disable Symbol \"DQMH_Disable_SEH\" to your project and set it to TRUE."
                  }
                }
                n115 = call-poly <vilib>:"Delacor_lib_QMH_Enqueue Message (poly).vi"("Priority Message? (F)"=TRUE, "Message"="Exit", "Message Queue in"=w262) -> ("error out"=w264:errorcluster)  [unwired: 7 in, 1 out]
              }
              frame True {
                # "If the module was launched externally, calling the Error Reported broadcast VI is the only action performed by the \"Error\" message. The module's caller can then process the error appropriately."
              }
            }
            n116 = Merge Errors(w257, w256) -> (w255:errorcluster)
          }
          frame "Exit" {
            w266 = -1073807346  # Session invalid.
            w281 = 91  # 91: not all Exit messages will have an argument
            w282 = TRUE  # Stop the VI
            # "Release the message queue reference"
            # "Exit - Exit the application."
            n117 = Variant To Data(error in=w288, type=T4 {"Module ID"=-1, "Origin"="", "Exit via Stop Module Req?"=FALSE, "Wait for Module to stop?"=FALSE} ("Stop Argument"), Variant=w280) -> (data=w277:T4, error out=w285:errorcluster)
            n118 = Unbundle By Name(w271) -> ("VISA resource"=w270:refnum<visa-resource-name>)
            n119 = call <vilib>:"Clear Errors.vi"("error in (no error)"=w285, "specific error code to clear (0: all)"=w281) -> ("error out"=w287:errorcluster)  [unwired: 4 in, 1 out]
            n120 = call-dynamic "Delacor_lib_QMH_Release Message Queue.vi"("error in"=w287, "Message Queue"=w283) -> ("error out"=w269:errorcluster)  [unwired: 9 in]
            n121 = VISA Clear(VISA resource name=w270, error in (no error)=w269) -> (VISA resource name out=w272:refnum<visa-resource-name>, error out=w273:errorcluster)
            n122 = call <vilib>:"Clear Errors.vi"("error in (no error)"=w273, "specific error code to clear (0: all)"=w266) -> ("error out"=w267:errorcluster)  [unwired: 4 in, 1 out]
            n123 = property on="Property Node" class="Mod Admin"(reference=w275) -> ("Accessors:Module ID"=w274:i32)  [unwired: 1 in, 2 out]
            n124 = control-ref of="This VI"() -> (w276:refnum<vi>)
            n125 = VISA Close(VISA resource name=w272, error in (no error)=w267) -> (error out=w268:errorcluster)
            n126 = call "Handle Exit.vi"("Stop Argument"=w277, "Module Admin in"=w275, "VI reference"=w276) -> ("error out"=w286:errorcluster, "Wait for Stop?"=w278:bool)  [unwired: 7 in]
            n127 = Merge Errors(w268, w286) -> (w284:errorcluster)
            n128 = call "Error Reported.vi"("Error"=w284, "Module ID"=w274) -> ()  [unwired: 9 in, 1 out]
          }
          frame Default {
            # "'Default' case only runs if there is a message that isn't defined in any of the other cases.  Output a programming error."
            n129 = property on="Property Node" class="Mod Admin"(reference=w296) -> ("Accessors:Module ID"=w295:i32)  [unwired: 1 in, 2 out]
            n130 = call "Module Name--constant.vi"("Module ID"=w295) -> ("Module Name"=w289:string)  [unwired: 10 in]
            n131 = Format Into String(format string="The invalid message string \"%s\" was received in the Message Handling Loop for module \"%s\".", w290, w289) -> (resulting string=w292:string)  [unwired: 2 in, 1 out]
            n132 = call <vilib>:"Error Cluster From Error Code.vi"("show call chain? (False)"=TRUE, "error message (\"\")"=w292, "error code (0)"=1) -> ("error out"=w298:errorcluster)  [unwired: 6 in]
            n133 = Merge Errors(w299, w298) -> (w300:errorcluster)
          }
          frame "Disconnect" {
            # "Request to disconnect from Arduino device."
            n134 = Variant To Data(error in=w310, type=T7 {"Module ID"=-1, "Boolean"=FALSE} ("Disconnect Argument"), Variant=w309) -> (data=w307:T7, error out=w303:errorcluster)
            n135 = Unbundle By Name(w307) -> ("Module ID"=w301:i32)
            n136 = Unbundle By Name(w306) -> ("VISA resource"=w305:refnum<visa-resource-name>, "Connected?"=w304:bool)
            n137 = case shown="False" w304 {
              tunnel: [w312 w318] -> w302
              tunnel: w305 -> [_ w322]
              tunnel: w303 -> [w313 w320]
              tunnel: w301 -> [w314 w317]
              frame False {
                n138 = Format Into String(format string="Module %d cannot disconnect from device. It was not connected." ("message"), w314) -> (resulting string=w311:string)  [unwired: 2 in, 1 out]
                n139 = call "Status Updated.vi"("error in"=w313, "Status"=w311, "Module ID"=w314) -> ("error out"=w312:errorcluster)  [unwired: 8 in]
              }
              frame True {
                n140 = VISA Clear(VISA resource name=w322, error in (no error)=w320) -> (VISA resource name out=w321:refnum<visa-resource-name>, error out=w323:errorcluster)
                n141 = VISA Close(VISA resource name=w321, error in (no error)=w323) -> (error out=w319:errorcluster)
                n142 = call "Device disconnected.vi"("error in"=w319, "Connected?"=FALSE, "Module ID"=w317) -> ("error out"=w318:errorcluster)  [unwired: 8 in]
              }
            }
          }
          frame "Init motors" {
            # "Request to initialize motors based on configuration paramerters."
            n143 = Variant To Data(error in=w336, type=T8 {"Module ID"=-1, "Comando"={"Action"=0, "Steps per rev motor 1"=0, "Steps per rev motor 2"=0, "RPM motor 1"=0, "RPM motor 2"=0}} ("Init motors Argument"), Variant=w335) -> (data=w333:T8, error out=w328:errorcluster)
            n144 = Unbundle By Name(w332) -> ("VISA resource"=w329:refnum<visa-resource-name>, "Connected?"=w331:bool)
            n145 = Unbundle By Name(w333) -> ("Comando"=w330:T9, "Module ID"=w324:i32)
            n146 = case shown="True" w331 {
              tunnel: w329 -> [_ w357]
              tunnel: [w343 w350] -> w327
              tunnel: w330 -> [_ w366]
              tunnel: w328 -> [w344 w352]
              tunnel: w324 -> [w342 _]
              tunnel: [_ w348] -> w325
              frame False {
                n147 = Format Into String(format string="Module %d cannot initiliaze motor. It is not connected." ("message"), w342) -> (resulting string=w345:string)  [unwired: 2 in, 1 out]
                n148 = call "Status Updated.vi"("error in"=w344, "Status"=w345, "Module ID"=w342) -> ("error out"=w343:errorcluster)  [unwired: 8 in]
              }
              frame True {
                w356 = T15 128 items=["Flush Receive Buffer"=16, "Write Transmit Buffer to Device"=32, "Flush Receive Buffer (No I/O)"=64, "Flush Transmit Buffer"=128] ("Mask")
                # "Add 1 to select positions to avoid sending null characters to port."
                # "Write initilization command. First element of cluster must be Initialize."
                n149 = Type Cast(x=w366) -> (*(type *) &x=w355:string)  [unwired: 1 in]
                n150 = VISA Flush I/O Buffer(VISA resource name=w357, mask (16)=w356, error in (no error)=w352) -> (VISA resource name out=w347:refnum<visa-resource-name>, error out=w358:errorcluster)
                n151 = Concatenate Strings(w355, "\r\n") -> (w354:string)
                n152 = Unflatten From String(type=u8[] [], binary string=w354, data includes array or string size? (T)=FALSE, error in (no error)=w358) -> (value=w360:u8[], error out=w361:errorcluster)  [unwired: 1 in, 1 out]
                n153 = Add(x=w360, y=u8[] [1, 0, 0, 1, 1, 1, 1]) -> (x+y=w362:u8[])
                n154 = Type Cast(x=w362) -> (*(type *) &x=w359:string)  [unwired: 1 in]
                n155 = VISA Write(VISA resource name=w347, write buffer=w359, error in (no error)=w361) -> (VISA resource name out=w349:refnum<visa-resource-name>, error out=w351:errorcluster)  [unwired: 1 out]
                n156 = call "Wait for motor init.vi"("error in (no error)"=w351, "VISA Refnum in"=w349) -> ("error out"=w350:errorcluster, "Motors ready?"=w348:bool)  [unwired: 7 in, 1 out]
              }
            }
            n157 = case shown="True" w325 {
              selector: w325 -> [_ w338]
              tunnel: w327 -> [w337 w341]
              tunnel: [w337 w340] -> w326
              tunnel: w324 -> [_ w339]
              frame False {
              }
              frame True {
                n158 = call "Motors ready.vi"("error in"=w341, "Motors ready?"=w338, "Module ID"=w339) -> ("error out"=w340:errorcluster)  [unwired: 8 in]
              }
            }
          }
          frame "Home motors" {
            # "Request to move motors to home position. Home position can be especified for each motor."
            n159 = Variant To Data(error in=w377, type=T10 {"Module ID"=-1, "Home direction (M1)"=1, "Home direction (M2)"=1} ("Home motors Argument"), Variant=w376) -> (data=w374:T10, error out=w368:errorcluster)
            n160 = Unbundle By Name(w374) -> ("Home direction (M1)"=w370:T11, "Home direction (M2)"=w369:T11)  [unwired: 1 out]
            n161 = Unbundle By Name(w373) -> ("Connected?"=w372:bool, "VISA resource"=w371:refnum<visa-resource-name>)
            n162 = case shown="True" w372 {
              tunnel: w371 -> [_ w385]
              tunnel: [w378 w391] -> w367
              tunnel: w370 -> [_ w388]
              tunnel: w369 -> [_ w381]
              tunnel: w368 -> [w378 w379]
              frame False {
              }
              frame True {
                n163 = Flatten To String(anything=w381, prepend array or string size? (T)=FALSE, error in (no error)=w379) -> (data string=w380:string, error out=w382:errorcluster)  [unwired: 1 in, 1 out]
                n164 = Flatten To String(anything=w388, prepend array or string size? (T)=FALSE, error in (no error)=w382) -> (data string=w387:string, error out=w389:errorcluster)  [unwired: 1 in, 1 out]
                n165 = Concatenate Strings("H", w387, w380) -> (w384:string)
                n166 = VISA Write(VISA resource name=w385, write buffer=w384, error in (no error)=w389) -> (error out=w391:errorcluster)  [unwired: 2 out]
              }
            }
          }
        }
        n167 = call-dynamic "Delacor_lib_QMH_Error Handler - Message Handling Loop.vi"("error in"=w170, "Message Queue in"=w161) -> ("dup error in"=w167:errorcluster)  [unwired: 8 in, 1 out]
      }
    }
    frame Error {
      n168 = call "Synchronize Caller Events.vi"("Module Admin"=w395) -> ("Module Admin out"=w394:refnum<class "Delacor_lib_QMH_Cloneable Module Admin.lvclass">)  [unwired: 9 in, 1 out]
      n169 = property on="Property Node" class="Mod Admin"(reference=w394) -> ("Accessors:Module ID"=w393:i32)  [unwired: 1 in, 2 out]
      n170 = call-dynamic "Delacor_lib_QMH_Release Message Queue.vi"("error in"=w401, "Message Queue"=w392) -> ("error out"=w400:errorcluster)  [unwired: 9 in]
      n171 = call "Module Name--constant.vi"("Module ID"=w393) -> ("Module Name"=w398:string)  [unwired: 10 in]
      n172 = Format Into String(format string="An error occurred during initialization. %s is no longer running.", w398) -> (resulting string=w396:string)  [unwired: 2 in, 1 out]
      n173 = call "Error Reported.vi"("Additional Information"=w396, "Error"=w400, "Module ID"=w393) -> ()  [unwired: 8 in, 1 out]
    }
  }
  n174 = Merge Errors(w17, w16) -> (w18:errorcluster)
  n175 = call "Close Module.vi"("error in"=w18, "Wait for stop?"=w2, "Module Admin in"=w4) -> ("error out"=w14:errorcluster, "External Launch"=w1:bool, "Module Admin out"=w3:refnum<class "Delacor_lib_QMH_Cloneable Module Admin.lvclass">)  [unwired: 6 in]
  n176 = Unregister For Events(event registration refnum=w9, error in=w14) -> (error out=w13:errorcluster)
  "error out" <- w13
  n177 = local write "Module Admin"(w3) -> ()
  n178 = case "External Launch?" shown="True" w1 {
    tunnel: w13 -> [_ w402]
    frame False {
    }
    frame True {
      n179 = case shown="No Error" w402 {
        frame No Error {
          n180 = invoke class="VI" method="FP.Close"() -> ()  [unwired: 3 in, 3 out]
        }
        frame Error {
          n181 = invoke class="VI" method="FP.Open"("Activate"=TRUE ("Activate?")) -> ()  [unwired: 4 in, 5 out]
        }
      }
    }
  }
